vi "9609 Value undefined for key--error.vi"(8 "error in":errorcluster, 11 "key":string) -> (0 "error out":errorcluster)   [LabVIEW 2024, in "Electronic Datasheet.lvlib"]
uses:
  Electronic Datasheet.lvlib
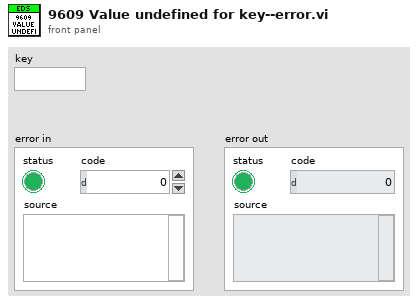
[diagram p1: front panel]
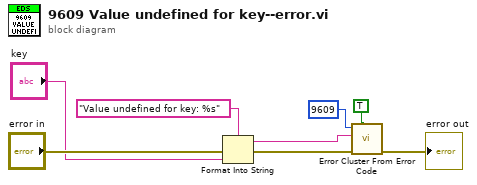
[diagram p0: block diagram]
diagram:
  n1 = Format Into String(format string="Value undefined for key: %s" ("error message (\"\")"), error in="error in", "key") -> (resulting string=w3:string, error out=w4:errorcluster)  [unwired: 1 in]
  n2 = call <vilib>:"Error Cluster From Error Code.vi"("show call chain? (False)"=TRUE, "error in (no error)"=w4, "error message (\"\")"=w3, "error code (0)"=9609) -> ("error out"=→"error out":errorcluster)  [unwired: 5 in]
